vi "sieve_of_eratosthenes.vi"() -> ()   [LabVIEW 2019]
panel:
  out "Took [ms]":u32
  out "Primes":i32[](array[numeric])
  out "Number of Primes":i32
  in  "Calc. primes up to":i32
  # "Lookup Table\n\n10              4\n100             25\n1000            168\n10_000          1229\n100_000         9592\n1_000_000       78498\n10_000_000      664579\n100_000_000     5761455"
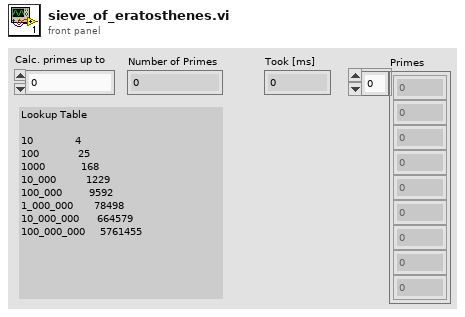
[diagram p1: front panel]
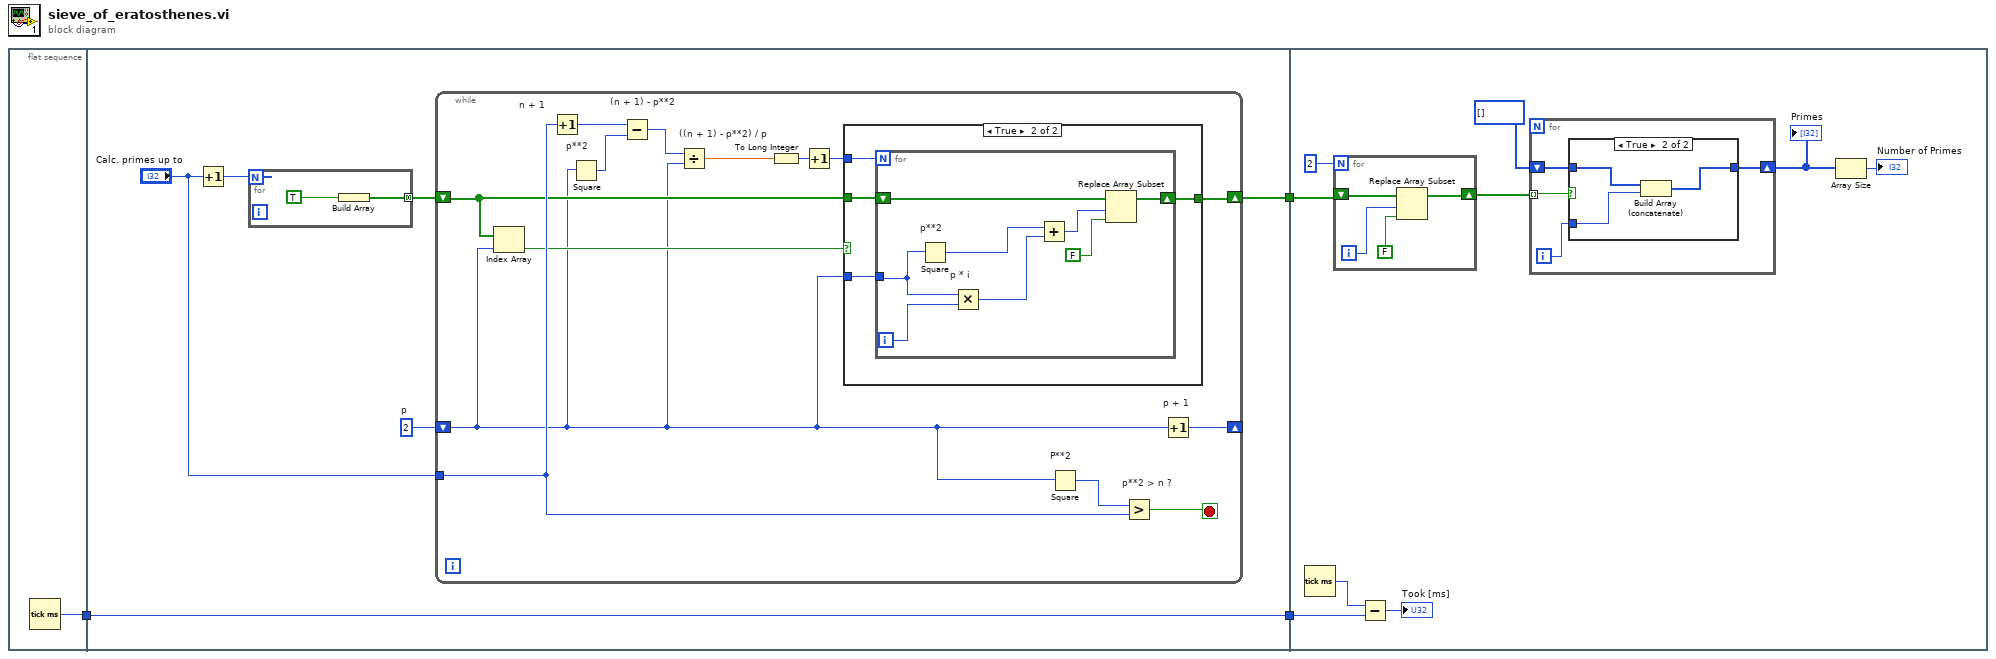
[diagram p0: block diagram]
diagram:
  n1 = flat-sequence {
    tunnel: [w4] -> w3
    tunnel: w3 -> [w5]
    tunnel: [w6] -> w2
    tunnel: [w5] -> w1
    tunnel: w2 -> [w40]
    tunnel: w1 -> [w43]
    frame #0 {
      n2 = Tick Count (ms)() -> (millisecond timer value=w4:u32)
    }
    frame #1 {
      w8 = 2  # p
      n3 = Increment(x="Calc. primes up to") -> (x+1=w10:i32)
      n4 = for {
        N: w10 -> [_]
        tunnel: [w38] -> w7 mode=concatenating
        n5 = Build Array(TRUE) -> (w38:bool[])
      }
      n6 = while {
        tunnel: "Calc. primes up to" -> [w22]
        shift-right: [w23] -> _
        shift-left: w8 -> [w14]
        shift-right: [w19] -> w6
        shift-left: w7 -> [w20]
        stop <- w11 stop-if-true
        n7 = Index Array(array=w20, index=w14) -> (element=w21:bool)
        n8 = Increment "n + 1"(x=w22) -> (x+1=w18:i32)
        n9 = Square "p**2"(x=w14) -> (x^2=w17:i32)
        n10 = Subtract "(n + 1) - p**2"(x=w18, y=w17) -> (x-y=w15:i32)
        n11 = Divide "((n + 1) - p**2) / p"(x=w15, y=w14) -> (x/y=w16:dbl)
        n12 = To Long Integer(number=w16) -> (32bit integer=w13:i32)
        n13 = Increment(x=w13) -> (x+1=w12:i32)
        n14 = case shown="True" w21 {
          tunnel: w12 -> [_ w29]
          tunnel: w14 -> [_ w28]
          tunnel: w20 -> [w25 w27]
          tunnel: [w25 w26] -> w19
          frame False {
          }
          frame True {
            n15 = for {
              N: w29 -> [_]
              tunnel: w28 -> [w33]
              shift-right: [w34] -> w26
              shift-left: w27 -> [w36]
              i -> [w37]
              n16 = Square "p**2"(x=w33) -> (x^2=w30:i32)
              n17 = Multiply "p * i"(x=w33, y=w37) -> (x*y=w31:i32)
              n18 = Add(x=w30, y=w31) -> (x+y=w32:i32)
              n19 = Replace Array Subset(array=w36, new element=FALSE, index=w32) -> (w34:bool[])
            }
          }
        }
        n20 = Square "P**2"(x=w14) -> (x^2=w24:i32)
        n21 = Greater? "p**2 > n ?"(x=w24, y=w22) -> (0:w11:bool)
        n22 = Increment "p + 1"(x=w14) -> (x+1=w23:i32)
      }
    }
    frame #2 {
      n23 = Tick Count (ms)() -> (millisecond timer value=w47:u32)
      n24 = for {
        N: 2 -> [_]
        shift-right: [w59] -> w46
        shift-left: w40 -> [w60]
        i -> [w58]
        n25 = Replace Array Subset(array=w60, new element=FALSE, index=w58) -> (w59:bool[])
      }
      n26 = Subtract(x=w47, y=w43) -> (x-y=→"Took [ms]":u32)
      n27 = for {
        tunnel: w46 -> [w51] mode=indexing
        shift-right: [w50] -> w44
        shift-left: i32[] [] -> [w49]
        i -> [w52]
        n28 = case shown="True" w51 {
          tunnel: w52 -> [_ w54]
          tunnel: [w53 w56] -> w50
          tunnel: w49 -> [w53 w55]
          frame False {
          }
          frame True {
            n29 = Build Array (concatenate)(w55, w54) -> (w56:i32[])
          }
        }
      }
      "Primes" <- w44
      n30 = Array Size(array=w44) -> (size(s)=→"Number of Primes":i32)
    }
  }
